vi "Net ID to Array.vi"(10 "Error In":errorcluster, 11 "Net ID":string) -> (2 "Error Out":errorcluster, 3 "Net ID (Array)":u8[](array[numeric]))   [LabVIEW 2016, in "TwinCAT ADS.lvlib"]
uses:
  TwinCAT ADS.lvlib
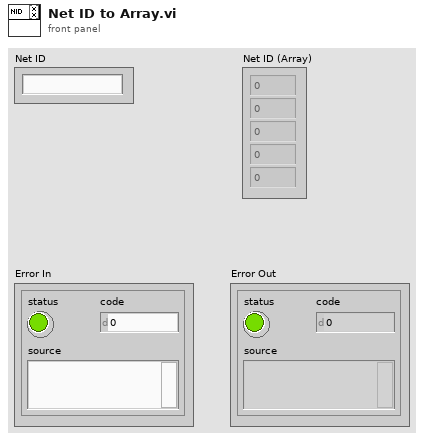
[diagram p1: front panel]
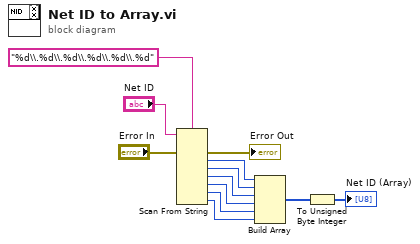
[diagram p0: block diagram]
diagram:
  n1 = Scan From String(format string="%d\\.%d\\.%d\\.%d\\.%d\\.%d", input string="Net ID", error in="Error In") -> (error out=→"Error Out":errorcluster, output 1=w5:i32, output 2=w6:i32, output 3=w7:i32, output 4=w8:i32, output 5=w9:i32, output 6=w10:i32)  [unwired: 7 in, 2 out]
  n2 = Build Array(w5, w6, w7, w8, w9, w10) -> (w11:i32[])
  n3 = To Unsigned Byte Integer(number=w11) -> (unsigned 8bit integer=→"Net ID (Array)":u8[])
